vi "Tell Reply.vi"(4 "Priority":bool, 7 "Actor in":refnum<class "Actor.lvclass">, 10 "Msg":refnum<class "Msg.lvclass">) -> (0 "Error out":errorcluster)   [LabVIEW 2025, in "jettl.lvlib"]
uses:
  jettl.lvlib
  Error/Error.lvlib
  Teller/Teller/Teller.lvclass
  Msg/Msg.lvclass
  Attributes/Attributes/Attributes.lvclass
  Actor/Actor.lvclass
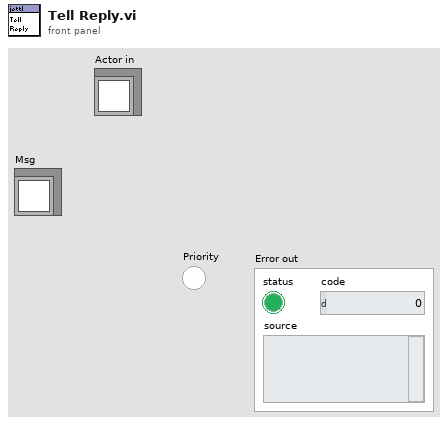
[diagram p1: front panel]
types:
  T1 = typedef "jettl.lvlib/Relation.ctl" = enum16{"Self", "Parent", "Child"}
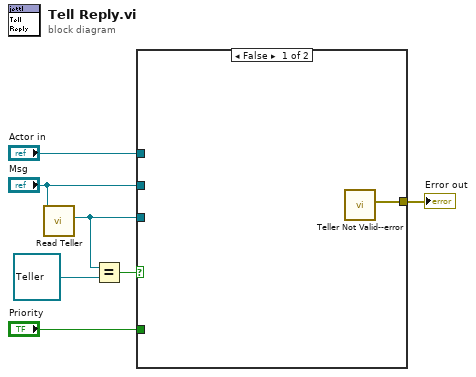
[diagram p0: block diagram]
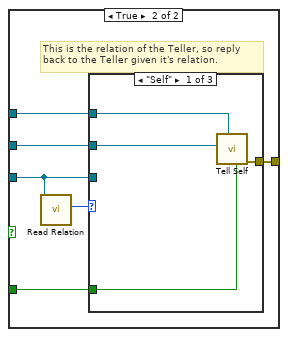
[diagram p2: hidden frame]
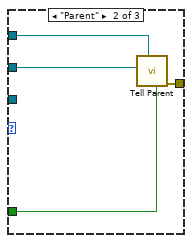
[diagram p3: hidden frame]
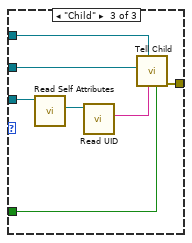
[diagram p4: hidden frame]
diagram:
  n1 = call-dynamic "Read Teller.vi"("Msg in"="Msg") -> ("Teller"=w2:refnum<class "Teller.lvclass">)  [unwired: 10 in]
  n2 = Equal?(x=w2, y=refnum<class "Teller.lvclass"> refnum ("Sender")) -> (x = y?=w5:bool)
  n3 = case shown="False" w5 {
    tunnel: "Actor in" -> [_ w14]
    tunnel: "Msg" -> [_ w13]
    tunnel: "Priority" -> [_ w12]
    tunnel: w2 -> [_ w11]
    tunnel: [w8 w9] -> w6
    frame False {
      n4 = call "Teller Not Valid--error.vi"() -> ("Error"=w8:errorcluster)  [unwired: 11 in]
    }
    frame True {
      # "This is the relation of the Teller, so reply back to the Teller given it's relation."
      n5 = call-dynamic "Read Relation.vi"("Teller in"=w11) -> ("Relation"=w10:T1)  [unwired: 10 in]
      n6 = case shown="\"Self\"" w10 {
        tunnel: w14 -> [w18 w22 w27]
        tunnel: w13 -> [w17 w21 w26]
        tunnel: w12 -> [w16 w20 w24]
        tunnel: w11 -> [_ _ w29]
        tunnel: [w15 w19 w23] -> w9
        frame "Self" {
          n7 = call "Tell Self.vi"("Priority"=w16, "Actor in"=w18, "Msg"=w17) -> ("Error out"=w15:errorcluster)  [unwired: 8 in]
        }
        frame "Parent" {
          n8 = call "Tell Parent.vi"("Priority"=w20, "Actor in"=w22, "Msg"=w21) -> ("Error out"=w19:errorcluster)  [unwired: 8 in]
        }
        frame "Child" {
          n9 = call-dynamic "Read Self Attributes.vi"("Teller in"=w29) -> ("Self Attributes"=w28:refnum<class "Attributes.lvclass">)  [unwired: 10 in]
          n10 = call-dynamic "Read UID.vi"("Attributes in"=w28) -> ("UID"=w25:string)  [unwired: 10 in]
          n11 = call "Tell Child.vi"("Priority"=w24, "UID"=w25, "Actor in"=w27, "Msg"=w26) -> ("Error out"=w23:errorcluster)  [unwired: 7 in]
        }
      }
    }
  }
  "Error out" <- w6
